vi "Vision Processing.vi"   [LabVIEW 2011]
doc: "This VI runs in parallel to other tasks. It gets images from the camera, processes them for color or shape and use that information to affect robot behavior."
uses:
  Robot Global Data.vi
types:
  T1 = typedef "Image Type" = u32
  T2 = typedef "WPI_CameraDevRef.ctl" = cluster{"Camera Address":string, "CameraStatus":errorcluster, "Acquire Image Notifier":refnum<notifier>}
  T3 = typedef "IMAQ Image.ctl" = refnum<image>
  T4 = typedef "WPI_CameraImageSize.ctl" = enum16{"640x480", "320x240", "160x120"}
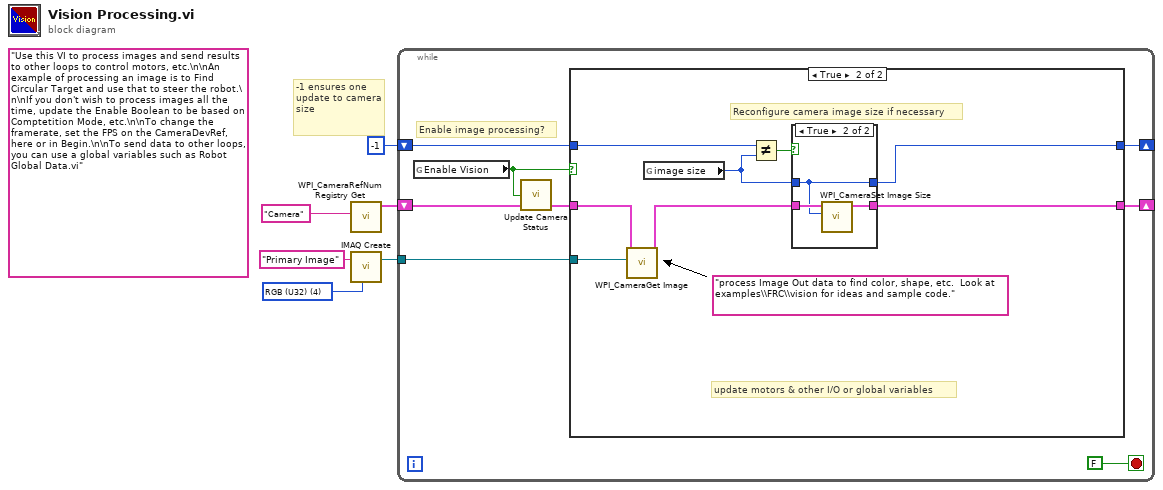
[diagram p0: block diagram]
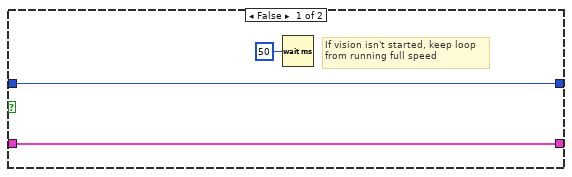
[diagram p2: hidden frame]
diagram:
  (unwired) "Use this VI to process images and send results to other loops to control motors, etc.\n\nAn example of processing an image is to Find Circular Target and use that to steer the robot.\n\nIf you don't wish to process images all the time, update the Enable Boolean to be based on Comptetition Mode, etc.\n\nTo change the framerate, set the FPS on the CameraDevRef, here or in Begin.\n\nTo send data to other loops, you can use a global variables such as Robot Global Data.vi"
  w6 = T1 4 items=["Grayscale (U8)", "Grayscale (I16)", "Grayscale (SGL)", "Complex (CSG)", "RGB (U32)", "HSL (U32)", "RGB (U64)"] ("Image Type")
  # "-1 ensures one update to camera size"
  n1 = call <vilib>:"WPI_CameraRefNum Registry Get.vi"("refnum name"="Camera") -> ("CameraDevRef"=w3:T2)  [unwired: 1 in, 9 out]
  n2 = call "IMAQ Create"("Image Name"="Primary Image", "Image Type"=w6) -> ("New Image"=w4:T3)  [unwired: 2 in, 2 out]
  n3 = while {
    shift-right: [w13] -> _
    shift-left: w3 -> [w11]
    tunnel: w4 -> [w12]
    shift-right: [w7] -> _
    shift-left: -1 -> [w8]
    stop <- FALSE stop-if-true
    # "Enable image processing?"
    n4 = global read "Robot Global Data.vi" "Enable Vision"() -> (w9:bool)
    n5 = call "Update Camera Status.vi"("CameraDevRef In"=w11, "Enable Vision"=w9) -> ("CameraDevRef Out"=w10:T2)  [unwired: 3 out]
    n6 = case shown="True" w9 {
      tunnel: w12 -> [_ w22]
      tunnel: [w17 w23] -> w13
      tunnel: w10 -> [w17 w19]
      tunnel: w8 -> [w15 w25]
      tunnel: [w15 w20] -> w7
      frame False {
        # "If vision isn't started, keep loop\nfrom running full speed"
        n7 = Wait (ms)(milliseconds to wait=u32 50) -> ()  [unwired: 1 out]
      }
      frame True {
        (unwired) "process Image Out data to find color, shape, etc.  Look at examples\\FRC\\vision for ideas and sample code."
        # "update motors & other I/O or global variables"
        # "Reconfigure camera image size if necessary"
        n8 = call <vilib>:"WPI_CameraGet Image.vi"("Image"=w22, "CameraDevRef"=w19) -> ("CameraDevRef Out"=w18:T2)  [unwired: 1 in, 8 out]
        n9 = global read "Robot Global Data.vi" "image size"() -> (w21:T4)
        n10 = Not Equal?(x=w25, y=w21) -> (x != y?=w24:bool)
        n11 = case shown="True" w24 {
          tunnel: w18 -> [w27 w30]
          tunnel: [w27 w29] -> w23
          tunnel: w21 -> [w26 w28]
          tunnel: [w26 w28] -> w20
          frame False {
          }
          frame True {
            n12 = call <vilib>:"WPI_CameraSet Image Size.vi"("Image Size"=w28, "CameraDevRef"=w30) -> ("CameraDevRef Out"=w29:T2)  [unwired: 1 in, 8 out]
          }
        }
      }
    }
  }
